vi "Avocent_build_command_toggle.vi"(10 "Set switches":bool[](array[boolean])=[FALSE, FALSE, FALSE, FALSE, FALSE, FALSE, FALSE, FALSE, FALSE, TRUE, FALSE, FALSE, FALSE, FALSE, FALSE, FALSE, FALSE, FALSE, FALSE, FALSE, FALSE, FALSE, FALSE, FALSE, FALSE, FALSE, FALSE, FALSE, FALSE, FALSE, FALSE, FALSE], 11 "Toggle On/Off":bool) -> (3 "HTTP Command":string="/3?3=admin,1234,0000000001000000,")   [LabVIEW 2013]
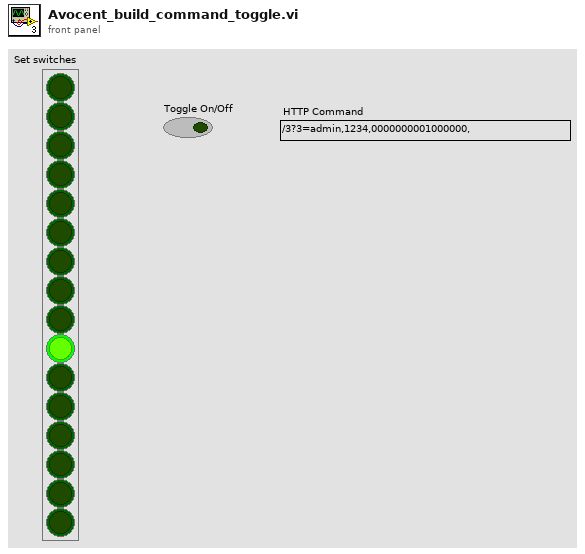
[diagram p1: front panel]
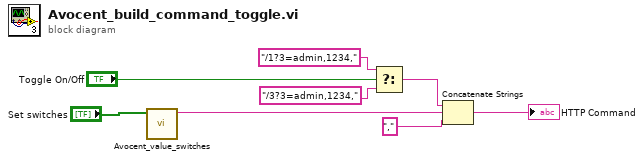
[diagram p0: block diagram]
diagram:
  n1 = call "Avocent_value_switches.vi"("Power indicator 2"="Set switches") -> ("spreadsheet string"=w7:string)  [unwired: 10 in]
  n2 = Select(t="/1?3=admin,1234," ("Command"), s="Toggle On/Off", f="/3?3=admin,1234," ("Command")) -> (s? t:f=w6:string)
  n3 = Concatenate Strings(w6, w7, "," ("Command")) -> (→"HTTP Command":string)
